vi "Configure Calibration Kit.vi"(7 "Connector type":T1(ring), 8 "error in (no error)":errorcluster, 10 "Cal kit Name":string, 11 "VNA-PNA in":refnum<class "VNA-PNA.lvclass">) -> (0 "error out":errorcluster, 3 "VNA-PNA out":refnum<class "VNA-PNA.lvclass">)   [LabVIEW 2020, in "VNA-PNA.lvclass"]
doc: "Configure the calibration kit to use."
uses:
  VNA-PNA.lvclass
  C:/Sandbox/Git_Sandbox/WiSpry Test Framework source code (LV20)/WiSpry Test Framework/Instruments/Instrument.lvclass
  Instrument.lvclass/Instrument.ctl
  Instrument.lvclass
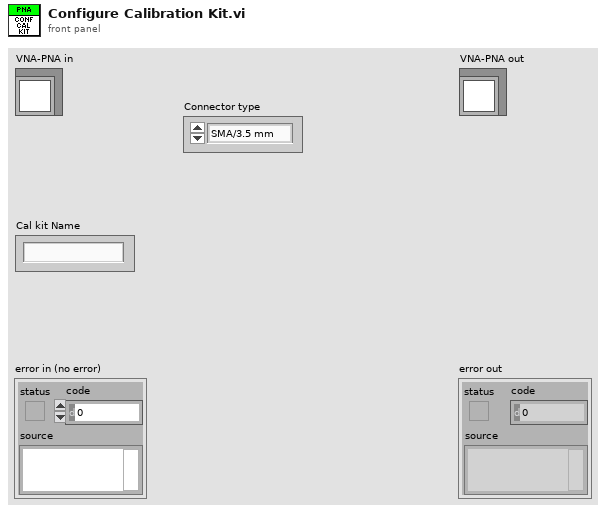
[diagram p1: front panel]
types:
  T1 = enum16{"SMA/3.5 mm", "2.92 mm", "2.4 mm", "1.85 mm", "N 50 Ohm", "N 75 Ohm", "7-16"}
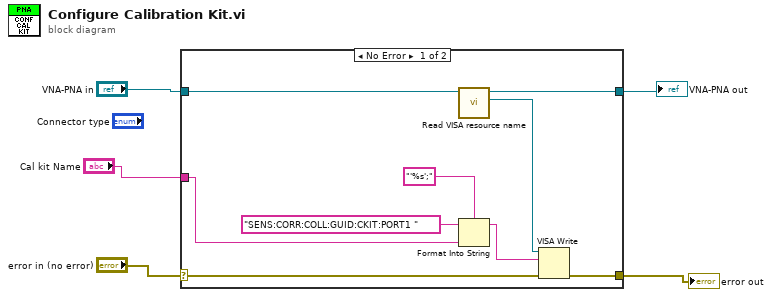
[diagram p0: block diagram]
diagram:
  n1 = case shown="No Error" "error in (no error)" {
    selector: "error in (no error)" -> [w13 w16]
    tunnel: "Cal kit Name" -> [w14 _]
    tunnel: [w12 w16] -> w2
    tunnel: "VNA-PNA in" -> [w11 w15]
    tunnel: [w10 w15] -> w1
    frame No Error {
      n2 = call "Read VISA resource name.vi"("Instrument in"=w11) -> ("VISA resource name"=w9:refnum<visa-resource-name>, "Instrument out"=w10:refnum<class "VNA-PNA.lvclass">)  [unwired: 9 in]
      n3 = Format Into String(format string="'%s';", initial string="SENS:CORR:COLL:GUID:CKIT:PORT1 ", w14) -> (resulting string=w6:string)  [unwired: 1 in, 1 out]
      n4 = VISA Write(VISA resource name=w9, write buffer=w6, error in (no error)=w13) -> (error out=w12:errorcluster)  [unwired: 2 out]
    }
    frame Error {
    }
  }
  "error out" <- w2
  "VNA-PNA out" <- w1
